vi "Post-Install Custom Action.vi"(10 "Variant":variant) -> (0 "error out":errorcluster)   [LabVIEW 2009]
uses:
  <vilib>/zip/NI_Unzip.lvlib
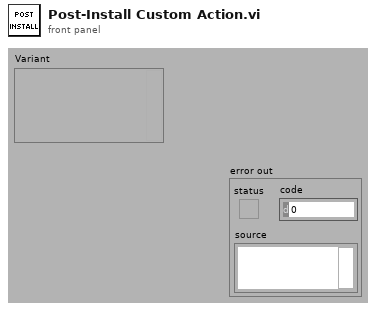
[diagram p1: front panel]
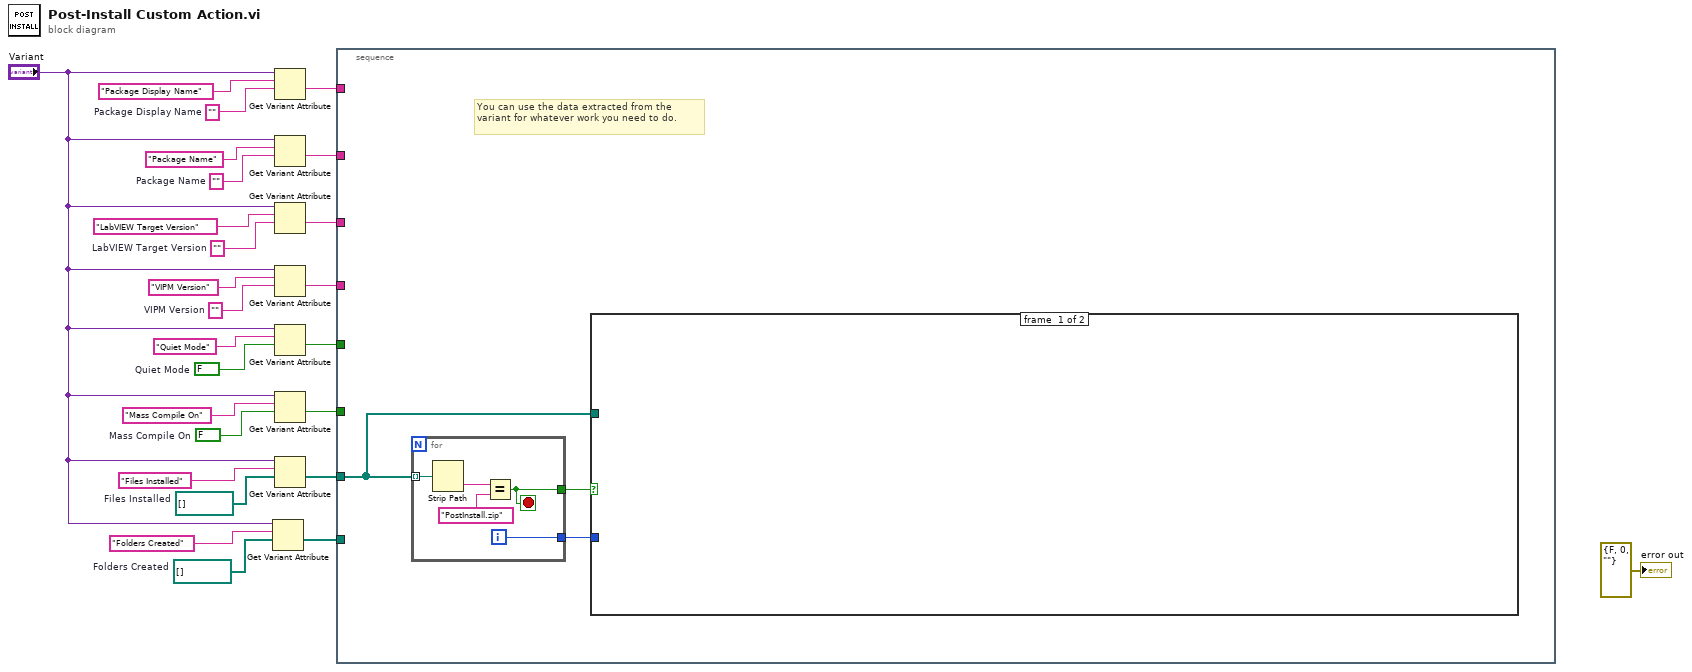
[diagram p0: block diagram]
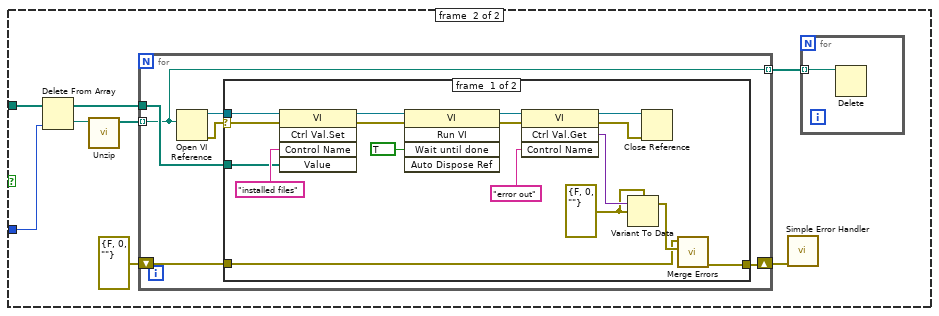
[diagram p2: hidden frame]
diagram:
  w1 = path[] []  # Folders Created
  w2 = path[] []  # Files Installed
  w8 = FALSE  # Mass Compile On
  w9 = ""  # Package Display Name
  w16 = FALSE  # Quiet Mode
  w19 = ""  # VIPM Version
  w21 = ""  # LabVIEW Target Version
  w23 = ""  # Package Name
  n1 = Get Variant Attribute(Variant="Variant", name="Folders Created", default value (empty Variant)=w1) -> (value=w6:path[])  [unwired: 1 in, 3 out]
  n2 = Get Variant Attribute(Variant="Variant", name="Package Display Name", default value (empty Variant)=w9) -> (value=w15:string)  [unwired: 1 in, 3 out]
  n3 = Get Variant Attribute(Variant="Variant", name="Package Name", default value (empty Variant)=w23) -> (value=w14:string)  [unwired: 1 in, 3 out]
  n4 = Get Variant Attribute(Variant="Variant", name="LabVIEW Target Version", default value (empty Variant)=w21) -> (value=w13:string)  [unwired: 1 in, 3 out]
  n5 = Get Variant Attribute(Variant="Variant", name="VIPM Version", default value (empty Variant)=w19) -> (value=w12:string)  [unwired: 1 in, 3 out]
  n6 = Get Variant Attribute(Variant="Variant", name="Quiet Mode", default value (empty Variant)=w16) -> (value=w11:bool)  [unwired: 1 in, 3 out]
  n7 = Get Variant Attribute(Variant="Variant", name="Mass Compile On", default value (empty Variant)=w8) -> (value=w10:bool)  [unwired: 1 in, 3 out]
  n8 = Get Variant Attribute(Variant="Variant", name="Files Installed", default value (empty Variant)=w2) -> (value=w5:path[])  [unwired: 1 in, 3 out]
  n9 = stacked-sequence {
    tunnel: w15 -> [_]
    tunnel: w14 -> [_]
    tunnel: w13 -> [_]
    tunnel: w12 -> [_]
    tunnel: w11 -> [_]
    tunnel: w10 -> [_]
    tunnel: w5 -> [w28]
    tunnel: w6 -> [_]
    frame #0 {
      # "You can use the data extracted from the variant for whatever work you need to do."
      n10 = for {
        tunnel: w28 -> [w67] mode=indexing
        tunnel: [w64] -> w29
        tunnel: [w63] -> w27
        i -> [w63]
        stop <- w64 stop-if-true
        n11 = Strip Path(path=w67) -> (name=w66:string)  [unwired: 1 out]
        n12 = Equal?(x=w66, y="PostInstall.zip") -> (x = y?=w64:bool)
      }
      n13 = case shown="True" w29 {
        tunnel: w28 -> [_ w37]
        tunnel: w27 -> [_ w36]
        frame #0 {
        }
        frame #1 {
          n14 = Delete From Array(array=w37, index=w36) -> (deleted portion=w35:path, array with subset deleted=w33:path[])  [unwired: 1 in]
          n15 = call <vilib>:"Unzip.vi"("Zip file"=w35) -> ("Unzipped files"=w34:path[])  [unwired: 8 in, 2 out]
          n16 = for {
            tunnel: w34 -> [w41] mode=indexing
            tunnel: w33 -> [w42]
            tunnel: [w41] -> w32 mode=indexing
            shift-right: [w40] -> w30
            shift-left: errorcluster {"status"=FALSE, "code"=0, "source"=""} ("error out") -> [w39]
            n17 = Open VI Reference(vi path=w41) -> (vi reference=w44:refnum<vi>, error out=w43:errorcluster)  [unwired: 5 in]
            n18 = case shown="No Error" w43 {
              selector: w43 -> [w58 _]
              tunnel: w44 -> [w61 _]
              tunnel: w42 -> [w59 _]
              tunnel: [w46 w62] -> w40
              tunnel: w39 -> [w45 w62]
              frame #0 {
                w48 = errorcluster {"status"=FALSE, "code"=0, "source"=""} ("error in")
                n19 = invoke class="VI" method="Ctrl Val.Set"(reference=w61, error in=w58, "Control Name"="installed files", "Value"=w59) -> (reference out=w57:refnum<vi>, error out=w56:errorcluster)  [unwired: 1 in, 3 out]
                n20 = invoke class="VI" method="Run VI"(reference=w57, error in=w56, "Wait until done"=TRUE ("Wait Until Done")) -> (reference out=w52:refnum<vi>, error out=w54:errorcluster)  [unwired: 2 in, 3 out]
                n21 = invoke class="VI" method="Ctrl Val.Get"(reference=w52, error in=w54, "Control Name"="error out") -> (reference out=w51:refnum<vi>, error out=w53:errorcluster, "Get Control Value Variant"=w49:variant)  [unwired: 1 in, 1 out]
                n22 = Variant To Data(error in=w48, Variant=w49, type=w48) -> (data=w47:errorcluster)  [unwired: 1 out]
                n23 = Close Reference(reference=w51, error in (no error)=w53) -> ()  [unwired: 1 out]
                n24 = call <vilib>:"Merge Errors.vi"("error in 2 (no error)"=w47, "error in 1 (no error)"=w45) -> ("error out"=w46:errorcluster)  [unwired: 5 in]
              }
              frame #1 {
              }
            }
          }
          n25 = call <vilib>:"Simple Error Handler.vi"("error in (no error)"=w30) -> ()  [unwired: 4 in, 5 out]
          n26 = for {
            tunnel: w32 -> [w38] mode=indexing
            n27 = Delete(path (use dialog)=w38) -> ()  [unwired: 4 in, 3 out]
          }
        }
      }
    }
  }
  "error out" <- errorcluster {"status"=FALSE, "code"=0, "source"=""} ("error out")
